vi "FPGA Main_SPI API - Solution.vi"() -> ()   [LabVIEW 2014]
uses:
  <userlib>/_NI SPI IP/FPGA/Controllers/Public/Transfer Settings.ctl
  <vilib>/Platform/TimedLoop/XDataNode/timing_clust.ctl
  <vilib>/Platform/TimedLoop/XDataNode/nitl_modes.ctl
  <vilib>/Platform/TimedLoop/XDataNode/wakeup.ctl
  <vilib>/SPI API/SPIAPI/DIO/SPI Digital IO Lines.ctl
  <vilib>/SPI API/SPIAPI/DIO/SPI DIO Enable Lines.ctl
  <vilib>/rvi/Emulation/niFpgaGetClockAttributes.vi
  <vilib>/rvi/Emulation/niFpgaSctlEmulationGetInTimedLoop.vi
  <vilib>/rvi/Emulation/niFpgaEmulationReportErrorSimple.vi
  <vilib>/rvi/Emulation/niFpgaCriticalErrorInLSC.vi
  <vilib>/Platform/TimedLoop/XDataNode/XDataNode.xnode
  <vilib>/Platform/TimedLoop/XDataNode/XDNodeRunTimeDep.lvlib
  <userlib>/_NI SPI IP/FPGA/Controllers/NI SPI IP FPGA.lvlib
panel:
  in  "SPI PHY Settings":T1={"Divide Value"=20, "Transfer Length (bits)"=32, "CS Asserted Polarity"=FALSE, "Clock Polarity (CPOL)"=FALSE, "Clock Phase (CPHA)"=FALSE, "Lengthen MISO Setup"=FALSE, "Direction Change Bit"=0, "MOSI Starts as Output"=FALSE, "Tristatable MOSI"=FALSE} {"Direction Change Bit" max=64 step=1; "Transfer Length (bits)" min=1 max=64 step=1}
  in  "Sample Rate (Hz)":u32=100000
  in  "Chip Select":u8
  in  "Tx":u64=2147483648 format="%b"
  out "Rx":u64(graph)
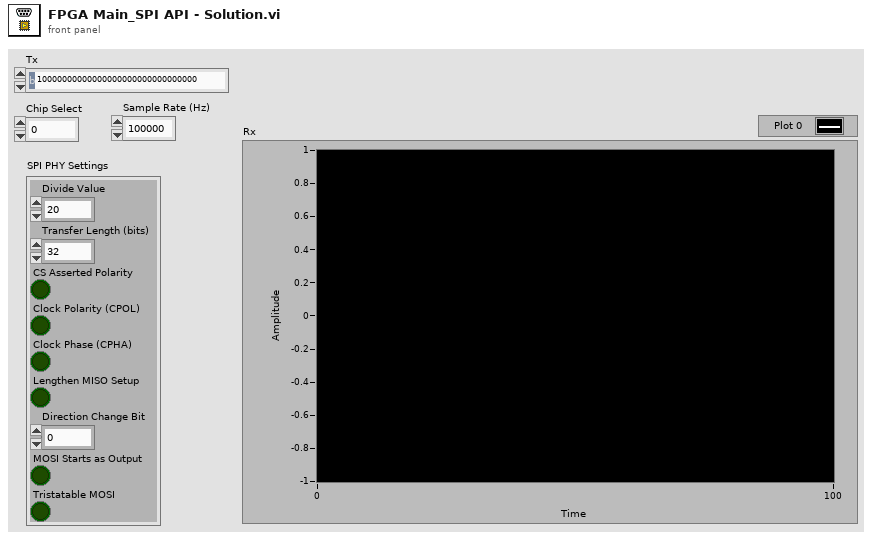
[diagram p1: front panel]
types:
  T1 = typedef "NI SPI IP FPGA.lvlib/Transfer Settings.ctl" = cluster{"Divide Value":u8, "Transfer Length (bits)":u8, "CS Asserted Polarity":bool, "Clock Polarity (CPOL)":bool, "Clock Phase (CPHA)":bool, "Lengthen MISO Setup":bool, "Direction Change Bit":u8, "MOSI Starts as Output":bool, "Tristatable MOSI":bool}
  T2 = typedef "SPI DIO Enable Lines.ctl" = cluster{"SCLK_en":refnum<k21>, "MISO_en":refnum<k21>, "MOSI_en":refnum<k21>, "CS0_en":refnum<k21>, "CS1_en":refnum<k21>, "CS2_en":refnum<k21>, "CS3_en":refnum<k21>, "CS4_en":refnum<k21>, "CS5_en":refnum<k21>}
  T3 = typedef "SPI Digital IO Lines.ctl" = cluster{"SCLK":refnum<k21>, "MISO":refnum<k21>, "MOSI":refnum<k21>, "CS 0":refnum<k21>, "CS 1":refnum<k21>, "CS 2":refnum<k21>, "CS 3":refnum<k21>, "CS 4":refnum<k21>, "CS 5":refnum<k21>}
  T4 = typedef "Internal Data (SPI API).ctl" = cluster{"DLU To SPI Engine Data FIFO":refnum<k21>, "SPI Engine to DLU Data FIFO":refnum<k21>, "Data to SPI Engine (Cache) Register":refnum<k21>, "SPI PHY Settings to SPI Engine (Cahche) Register":refnum<k21>}
  T5 = typedef "XDNodeRunTimeDep.lvlib/timing_clust.ctl" = cluster{"Expected End [f-1]":u64, "Actual End [f-1]":u64, "Finished Late? [f-1]":bool, "Expected End [i-1]":u64, "Actual End [i-1]":u64, "Finished Late? [i-1]":bool, "Expected Start [i]":u64, "Actual Start [i]":u64, "Expected Start [f]":u64, "Actual Start [f]":u64, "Source Name":string, "Structure Name":string, "Period":i64, "Deadline":i64, "Offset":i64, "Start":i64, "Priority":i32, "Timeout":i32, "Mode":T6, "Wakeup Reason":T7, "Error":errorcluster, "Source Type":string, "Secondary Source Type":string, "Global End Time":u64, "Global Start Time":u64, "Frame Duration":u64, "Iteration Duration":u64, "Assigned CPU":i32, "I/O Scan Engine Mode":u32}
  T6 = typedef "XDNodeRunTimeDep.lvlib/nitl_modes.ctl" = enum32{"No Change", "Process missed periods, maintain original phase", "Discard missed periods, maintain original phase", "Process missed periods, ignore original phase", "Discard missed periods, ignore original phase"}
  T7 = typedef "XDNodeRunTimeDep.lvlib/wakeup.ctl" = enum32{"Normal", "Aborted", "Asynchronous wakeup", "Timing source error", "Timed loop error", "Timeout"}
  T8 = typedef "SPI Response Information.ctl" = cluster{"Data to Node":u64, "Node Id":u16}
  T9 = typedef "NI SPI IP FPGA.lvlib/Spi Master Inputs.ctl" = cluster{"MISO":bool}
  T10 = typedef "NI SPI IP FPGA.lvlib/Spi Master Outputs.ctl" = cluster{"Chip Select":bool, "Clock":bool, "MOSI":bool, "MOSI OE":bool}
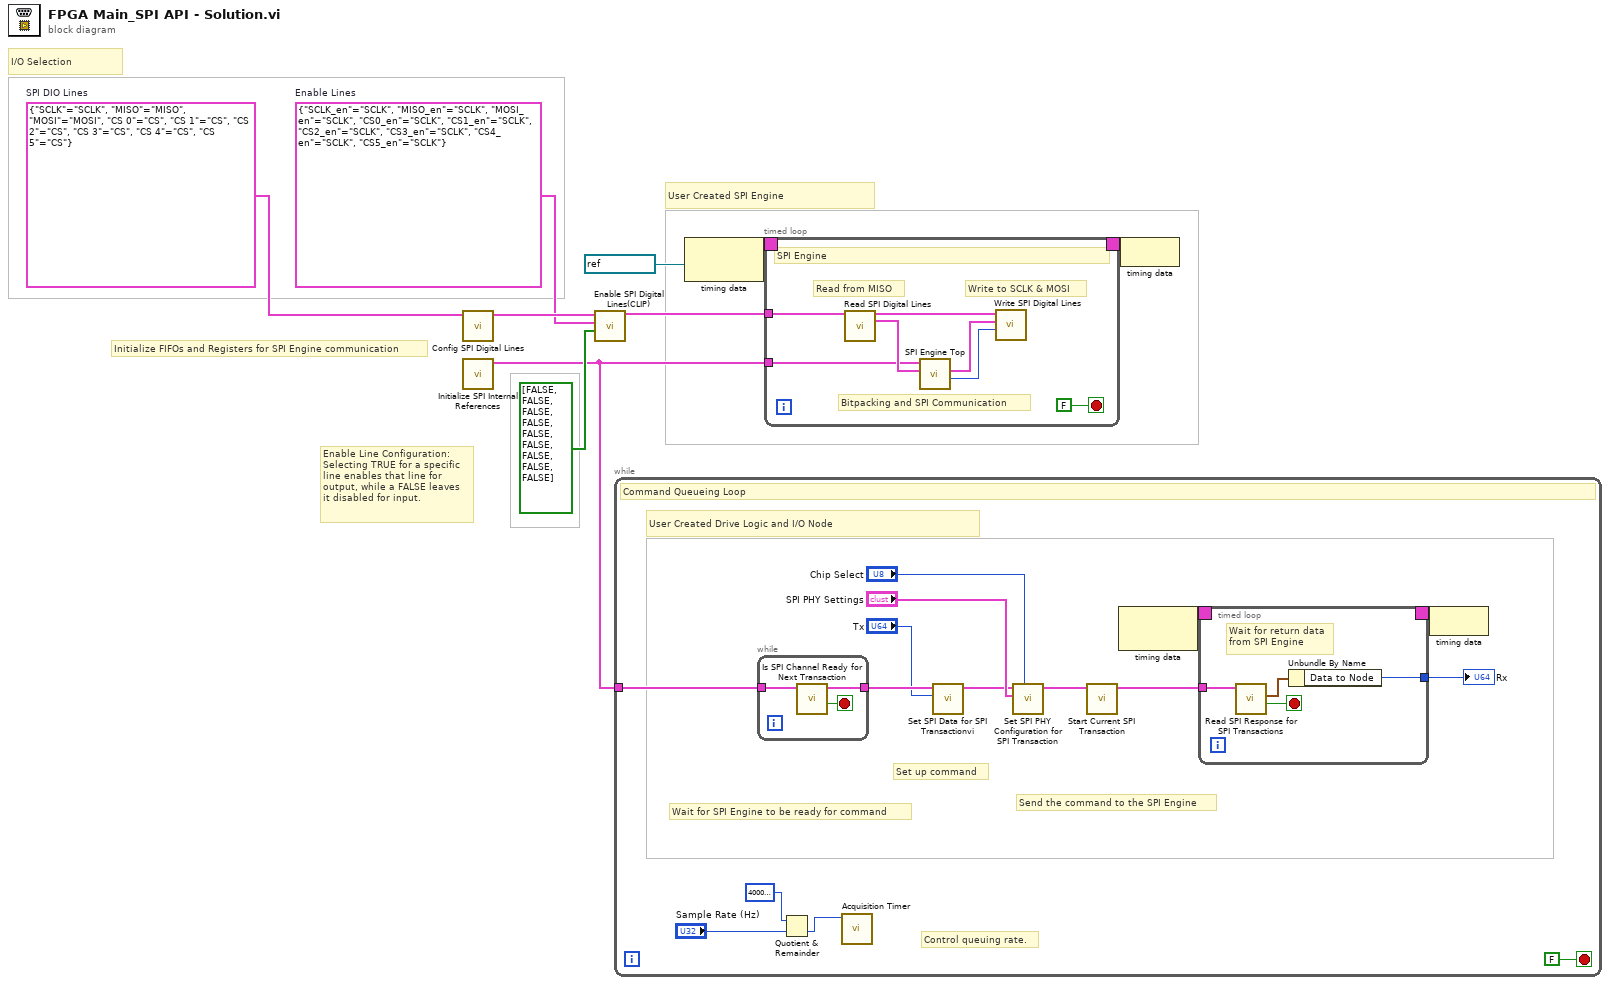
[diagram p0: block diagram]
diagram:
  w1 = T2 {"SCLK_en"="SCLK", "MISO_en"="SCLK", "MOSI_en"="SCLK", "CS0_en"="SCLK", "CS1_en"="SCLK", "CS2_en"="SCLK", "CS3_en"="SCLK", "CS4_en"="SCLK", "CS5_en"="SCLK"}  # Enable Lines
  w2 = T3 {"SCLK"="SCLK", "MISO"="MISO", "MOSI"="MOSI", "CS 0"="CS", "CS 1"="CS", "CS 2"="CS", "CS 3"="CS", "CS 4"="CS", "CS 5"="CS"}  # SPI DIO Lines
  # "I/O Selection"
  # "Initialize FIFOs and Registers for SPI Engine communication"
  # "Enable Line Configuration:\nSelecting TRUE for a specific\nline enables that line for\noutput, while a FALSE leaves\nit disabled for input."
  # "User Created SPI Engine"
  n1 = call <vilib>:"Config SPI Digital Lines.vi"("SPI DIO Lines"=w2) -> ("Chip Select DIO Lines"=w5:T3)  [unwired: 9 in, 1 out]
  n2 = call <vilib>:"Initialize SPI Internal References.vi"() -> ("SPI API References"=w3:T4)  [unwired: 10 in, 1 out]
  n3 = call <vilib>:"Enable SPI Digital Lines(CLIP).vi"("Enable"=bool[] [FALSE, FALSE, FALSE, FALSE, FALSE, FALSE, FALSE, FALSE, FALSE], "Enable Lines"=w1, "SPI DIO Lines"=w5) -> ("Chip Select DIO Lines"=w7:T3)  [unwired: 7 in, 1 out]
  n4 = while {
    tunnel: w3 -> [w16]
    stop <- FALSE stop-if-true
    # "Control queuing rate."
    # "Send the command to the SPI Engine"
    # "Set up command"
    # "Wait for SPI Engine to be ready for command"
    # "User Created Drive Logic and I/O Node"
    # "Command Queueing Loop"
    n5 = while {
      tunnel: w16 -> [w34]
      tunnel: [w33] -> w21
      stop <- w35 stop-if-true
      n6 = call <vilib>:"Is SPI Channel Ready for Next Transaction.vi"("Private Data In"=w34) -> ("SPI Channel Ready"=w35:bool, "Private Data Out"=w33:T4)  [unwired: 7 in, 2 out]
    }
    n7 = Quotient & Remainder(x=u32 40000000 ("Sample Rate (Hz)"), y="Sample Rate (Hz)") -> (floor(x/y)=w12:u32)  [unwired: 1 out]
    n8 = call <vilib>:"Acquisition Timer.vi"("Loop Time (Ticks)"=w12) -> ()  [unwired: 10 in, 1 out]
    n9 = call <vilib>:"Set SPI Data for SPI Transactionvi.vi"("Data In"="Tx", "Private Data In"=w21) -> ("Private Data Out"=w19:T4)  [unwired: 8 in, 1 out]
    n10 = call <vilib>:"Set SPI PHY Configuration for SPI Transaction.vi"("Chip Select"="Chip Select", "SPI PHY Settings"="SPI PHY Settings", "Private Data In"=w19) -> ("Private Data Out"=w18:T4)  [unwired: 7 in, 1 out]
    n11 = call <vilib>:"Start Current SPI Transaction.vi"("Private Data In"=w18) -> ("Private Data Out"=w17:T4)  [unwired: 8 in, 2 out]
    n12 = node-c288() -> (w24:T5)  [unwired: 1 in]
    n13 = timed-loop {
      timing: w24 -> [_]
      timing-out: [_] -> w23
      tunnel: w17 -> [w28]
      tunnel: [w25] -> w15
      stop <- w27 stop-if-true
      # "Wait for return data\nfrom SPI Engine"
      n14 = call <vilib>:"Read SPI Response for SPI Transactions.vi"("Private Data In"=w28) -> ("Read Data Valid?"=w27:bool, "Read Data"=w26:T8)  [unwired: 7 in, 2 out]
      n15 = Unbundle By Name(w26) -> ("Data to Node"=w25:u64)
    }
    "Rx" <- w15
    n16 = node-c288(w23) -> ()
  }
  n17 = node-c288(refnum<k21> "120MHz" ("Source Name")) -> (w9:T5)
  n18 = timed-loop {
    timing: w9 -> [_]
    timing-out: [_] -> w8
    tunnel: w7 -> [w38]
    tunnel: w3 -> [w36]
    stop <- FALSE stop-if-true
    # "Bitpacking and SPI Communication"
    # "Write to SCLK & MOSI"
    # "Read from MISO"
    # "SPI Engine"
    n19 = call <vilib>:"Read SPI Digital Lines.vi"("Chip Select DIO Lines"=w38) -> ("Chip Select DIO Lines Out"=w42:T3, "SPI Read Data"=w41:T9)  [unwired: 12 in, 1 out]
    n20 = call <vilib>:"SPI Engine Top.vi"("SPI Read Data"=w41, "SPI API References"=w36) -> ("Chip Select ID"=w39:u8, "SPI DIO Output"=w40:T10)  [unwired: 6 in, 2 out]
    n21 = call <vilib>:"Write SPI Digital Lines.vi"("CS Index"=w39, "spi output"=w40, "Chip Select DIO Lines"=w42) -> ()  [unwired: 7 in, 2 out]
  }
  n22 = node-c288(w8) -> ()
